vi "PH_Beckhoff.contents.vi"   [LabVIEW 2014, in "PH_Beckhoff.lvlib"]
doc: "This class is forseen to xxx\n\nThis class is part of the PHELIX xxx layer."
uses:
  PH_Beckhoff.lvlib
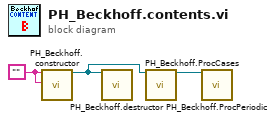
[diagram p0: block diagram]
diagram:
  w1 = ""
  n1 = call "PH_Beckhoff.constructor.vi"("name"=w1, "data in"=w1) -> ("i ref out"=w2:refnum<vi>)  [unwired: 15 in, 2 out]
  n2 = call "PH_Beckhoff.destructor.vi"("i ref in"=w2) -> ()  [unwired: 18 in, 1 out]
  n3 = call "PH_Beckhoff.ProcCases.vi"("i ref in"=w2) -> ("i ref out"=w3:refnum<vi>)  [unwired: 16 in, 2 out]
  n4 = call "PH_Beckhoff.ProcPeriodic.vi"("i ref in"=w3) -> ()  [unwired: 16 in, 3 out]
